vi "Module Loop.vi"(8 "error in (no error)":errorcluster, 11 "Config Updater Module in":refnum<class "Git Updater Module.lvclass">) -> (0 "error out":errorcluster, 3 "Config Updater Module out":refnum<class "Git Updater Module.lvclass">)   [LabVIEW 2020, in "Volatus.lvlib" / "Git Updater Module.lvclass"]
uses:
  Git Updater Module.lvclass
  C:/dev/lv20CE/relink/lv-volatus/Volatus/Module/Module.lvclass
  Module/Module.lvclass/Module.ctl
  Module/Module.lvclass
  MessageQ/MessageQ.lvclass/MessageQ.ctl
  MessageQ/Send.vi
  <vilib>/Utility/error.llb/Error Cluster From Error Code.vi
  Git Updater Module.lvclass/Git Updater Module.ctl
  Volatus.lvlib
panel:
  out "Tag":string
  out "Branch":string
  out "Hash":string
  # "Current Info"
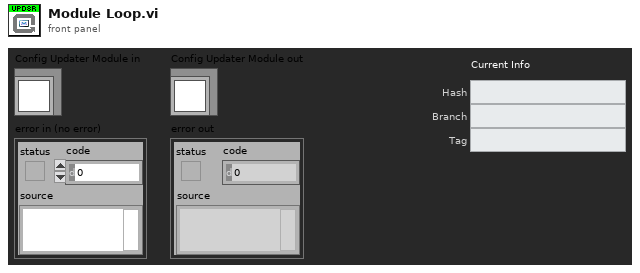
[diagram p1: front panel]
types:
  T1 = enum32{"Invalid", "Standard", "Closed", "Hidden", "Minimized", "Maximized"}
  T2 = typedef "Volatus.lvlib/Git Updater Module.lvclass/Git Info.ctl" = cluster{"Commit":string, "Branch":string, "Tag":string, "Branches":string[], "Tags":string[]}
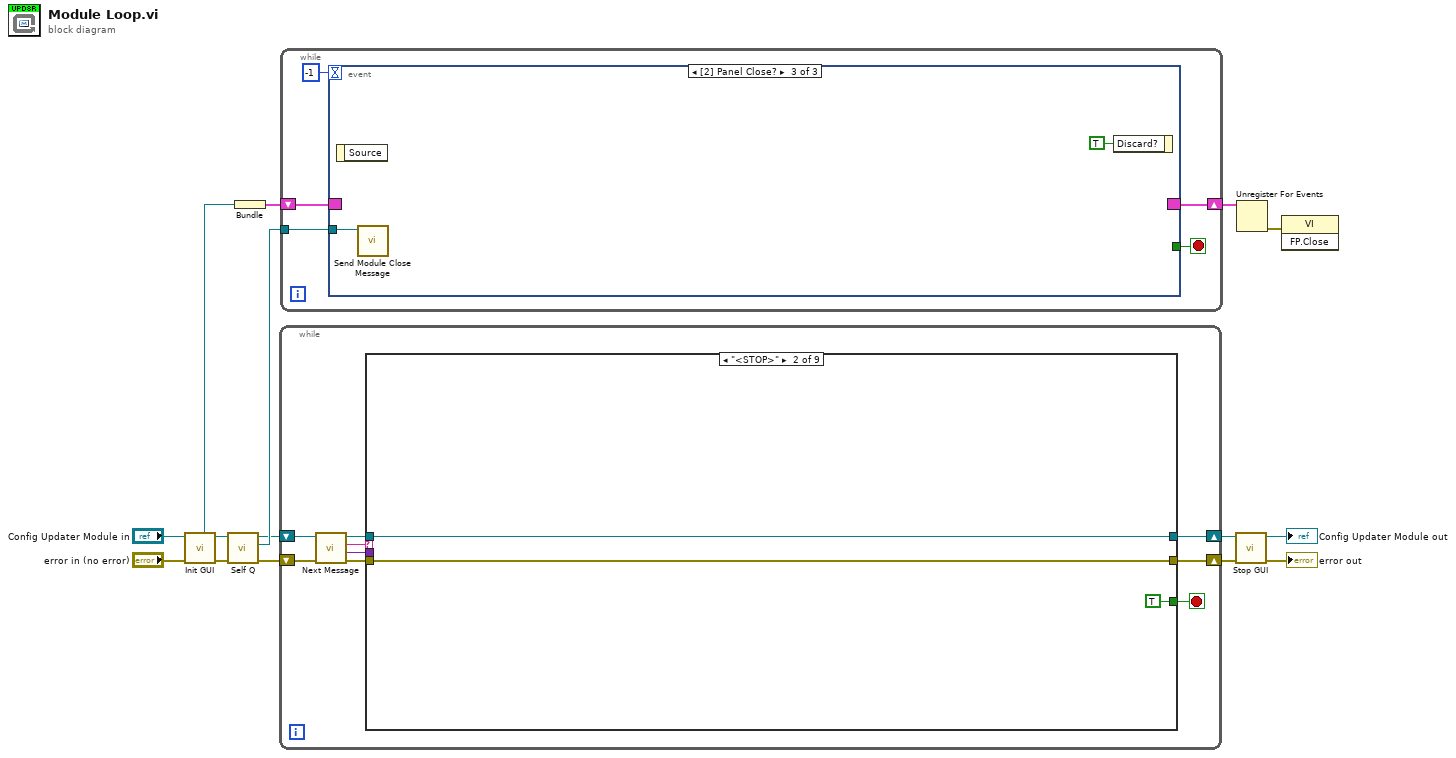
[diagram p0: block diagram]
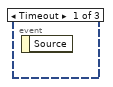
[diagram p2: hidden frame]
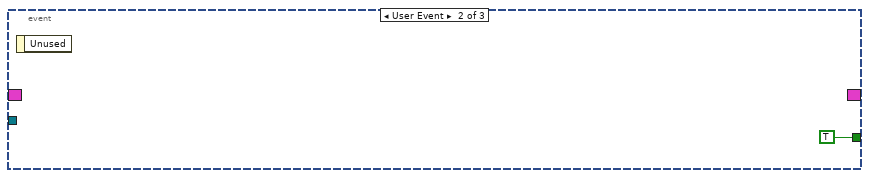
[diagram p3: hidden frame]
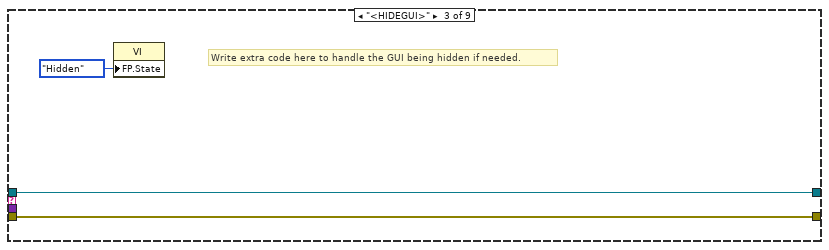
[diagram p5: hidden frame]
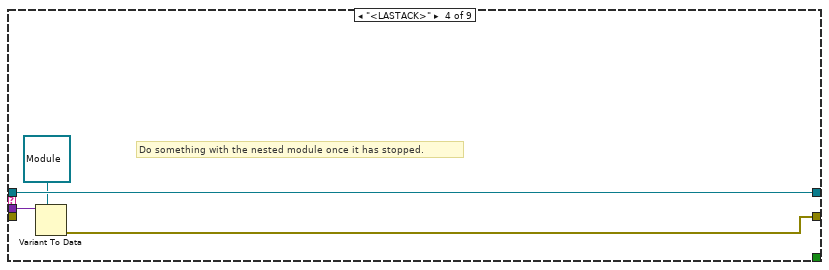
[diagram p6: hidden frame]
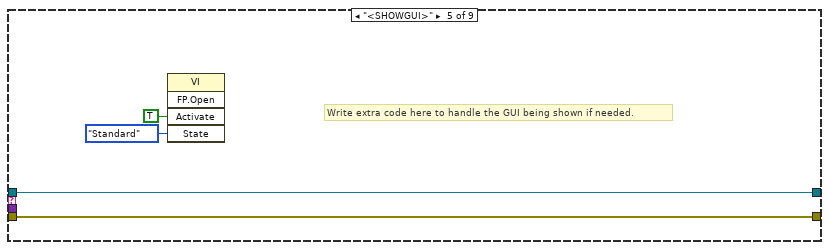
[diagram p7: hidden frame]
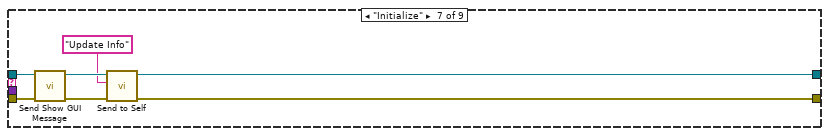
[diagram p9: hidden frame]
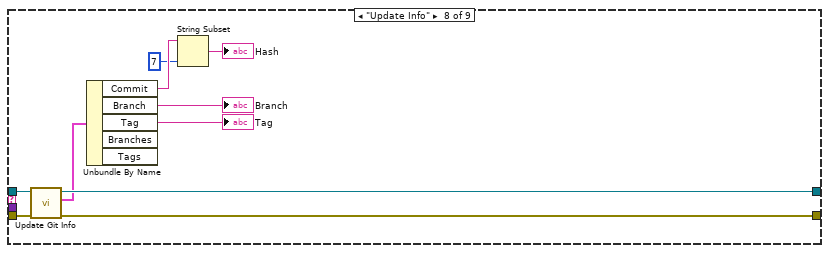
[diagram p10: hidden frame]
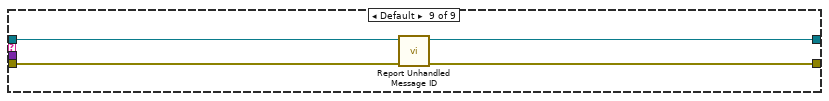
[diagram p11: hidden frame]
diagram:
  n1 = call "Init GUI.vi"("Module in"="Config Updater Module in") -> ("Module out"=w7:refnum<class "Git Updater Module.lvclass">, "Event Reg"=w12:refnum<event-registration>)  [unwired: 9 in]
  n2 = call "Self Q.vi"("Module in"=w7) -> ("Self Q"=w6:refnum<class "MessageQ.lvclass">, "Module out"=w5:refnum<class "Git Updater Module.lvclass">)  [unwired: 9 in]
  n3 = Bundle("Event Reg"=w12) -> (w8:cluster{"Event Reg":refnum<event-registration>})  [unwired: 1 in]
  n4 = while {
    shift-right: [w17] -> w10
    shift-left: w5 -> [w22]
    shift-right: [w16] -> w11
    shift-left: "error in (no error)" -> [w21]
    stop <- w15 stop-if-true
    n5 = call "Next Message.vi"("error in (no error)"=w21, "Module in"=w22) -> ("error out"=w20:errorcluster, "Data"=w14:variant, "ID"=w19:string, "Module out"=w18:refnum<class "Git Updater Module.lvclass">)  [unwired: 6 in]
    n6 = case shown="\"<STOP>\"" w19 {
      tunnel: w20 -> [w23 w26 w28 _ w37 w39 w47 w57 w61]
      tunnel: w18 -> [w24 w27 w29 w34 w38 w40 w45 w55 w59]
      tunnel: [w24 w27 w29 w34 w38 w40 w42 w54 w58] -> w17
      tunnel: [w23 w26 w28 w31 w37 w39 w44 w56 w60] -> w16
      tunnel: [_ TRUE _ _ _ _ _ _ _] -> w15
      tunnel: w14 -> [_ _ _ w33 _ _ _ _ _]
      frame "<CLOSE>" {
        # "If the module might be in a state that can be stopped, add logic to decide whether or not to actually stop."
        # "Add additional code to handle stopping the module."
      }
      frame "<STOP>" {
      }
      frame "<HIDEGUI>" {
        # "Write extra code here to handle the GUI being hidden if needed."
        n7 = property class="VI"("FP.State"=T1."Hidden" ("Front Panel Window:State")) -> ()  [unwired: 2 in, 2 out]
      }
      frame "<LASTACK>" {
        # "Do something with the nested module once it has stopped."
        n8 = Variant To Data(type=refnum<class "Module.lvclass"> refnum ("Volatus:Module"), Variant=w33) -> (error out=w31:errorcluster)  [unwired: 1 in, 1 out]
      }
      frame "<SHOWGUI>" {
        # "Write extra code here to handle the GUI being shown if needed."
        n9 = invoke class="VI" method="FP.Open"("Activate"=TRUE ("Activate?"), "State"=T1."Standard") -> ()  [unwired: 3 in, 5 out]
      }
      frame "<TIMEOUT>" {
        # "No message for this module was received in time"
      }
      frame "Initialize" {
        n10 = call "Send Show GUI Message.vi"("error in (no error)"=w47, "Module in"=w45) -> ("error out"=w46:errorcluster, "Module out"=w43:refnum<class "Git Updater Module.lvclass">)  [unwired: 8 in]
        n11 = call "Send to Self.vi"("error in (no error)"=w46, "Message ID"="Update Info", "Module in"=w43) -> ("error out"=w44:errorcluster, "Module out"=w42:refnum<class "Git Updater Module.lvclass">)  [unwired: 7 in]
      }
      frame "Update Info" {
        n12 = call "Update Git Info.vi"("error in (no error)"=w57, "Git Updater Module in"=w55) -> ("error out"=w56:errorcluster, "Git Info"=w53:T2, "Git Updater Module out"=w54:refnum<class "Git Updater Module.lvclass">)  [unwired: 7 in]
        n13 = Unbundle By Name(w53) -> ("Commit"=w52:string, "Branch"=→"Branch":string, "Tag"=→"Tag":string)  [unwired: 2 out]
        n14 = String Subset(string=w52, length (rest)=7 ("length (rest)")) -> (substring=→"Hash":string)  [unwired: 1 in]
      }
      frame Default {
        n15 = call "Report Unhandled Message ID.vi"("error in (no error)"=w61, "Module in"=w59) -> ("error out"=w60:errorcluster, "Module out"=w58:refnum<class "Git Updater Module.lvclass">)  [unwired: 8 in]
      }
    }
  }
  n16 = while {
    tunnel: w6 -> [w66]
    shift-right: [w64] -> w9
    shift-left: w8 -> [w65]
    stop <- w63 stop-if-true
    n17 = event shown="[2] Panel Close?" {
      selector: w65 -> [_ _ _]
      dyn-events: [_ _ _] -> w64
      timeout: -1 -> [_ _ _]
      tunnel: w66 -> [_ _ w68]
      tunnel: [_ TRUE _] -> w63
      event Timeout {
        n18 = event-data() -> ()  [unwired: 1 in, 1 out]
      }
      event User Event {
        n19 = event-data() -> ()  [unwired: 1 in, 1 out]
      }
      event Panel Close? {
        n20 = event-data() -> ()  [unwired: 1 in, 1 out]
        n21 = call "Send Module Close Message.vi"("MessageQ"=w68) -> ()  [unwired: 10 in, 1 out]
        n22 = event-data("Discard?"=TRUE) -> ()  [unwired: 1 in, 1 out]
      }
    }
  }
  n23 = call "Stop GUI.vi"("error in (no error)"=w11, "Module in"=w10) -> ("error out"=→"error out":errorcluster, "Module out"=→"Config Updater Module out":refnum<class "Git Updater Module.lvclass">)  [unwired: 8 in]
  n24 = Unregister For Events(event registration refnum=w9) -> (error out=w13:errorcluster)  [unwired: 1 in]
  n25 = invoke class="VI" method="FP.Close"(error in=w13) -> ()  [unwired: 2 in, 3 out]
